vi "Detect Fit Points.vi"(1 "Point Array B":T1, 2 "Point Array A":cluster{"X Values":dbl[], "Y Values":dbl[]}) -> (0 "False Data?":i32[](array[numeric]))   [LabVIEW 2017]
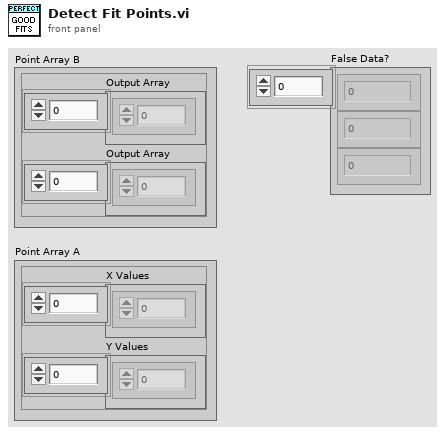
[diagram p1: front panel]
types:
  T1 = cluster{"Output Array":dbl[], "Output Array":dbl[]}
  T2 = cluster{"Starting Element":dbl, "Numeric Control":dbl}
  T3 = cluster{"Numeric Control":dbl, "Numeric Control":dbl}
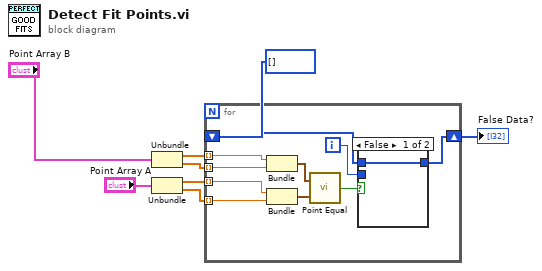
[diagram p0: block diagram]
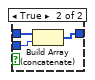
[diagram p2: hidden frame]
diagram:
  n1 = Unbundle("Point Array B") -> ("Output Array"=w3:dbl[], "Output Array"=w4:dbl[])
  n2 = Unbundle("Point Array A") -> ("X Values"=w5:dbl[], "Y Values"=w6:dbl[])
  n3 = for {
    tunnel: w3 -> [w18] mode=indexing
    tunnel: w4 -> [w17] mode=indexing
    tunnel: w5 -> [w14] mode=indexing
    tunnel: w6 -> [w13] mode=indexing
    shift-right: [w10] -> w7
    shift-left: i32[] [] -> [w9]
    i -> [w12]
    n4 = Bundle("Starting Element"=w18, "Numeric Control"=w17) -> (w16:T2)  [unwired: 1 in]
    n5 = Bundle("Numeric Control"=w14, "Numeric Control"=w13) -> (w15:T3)  [unwired: 1 in]
    n6 = call "Point Equal.vi"("Point B"=w15, "Point A"=w16) -> ("Equal"=w11:bool)
    n7 = case shown="False" w11 {
      tunnel: w12 -> [_ w22]
      tunnel: [w19 w21] -> w10
      tunnel: w9 -> [w19 w20]
      frame False {
      }
      frame True {
        n8 = Build Array (concatenate)(w20, w22) -> (w21:i32[])
      }
    }
  }
  "False Data?" <- w7
